vi "All GEMM.vi"() -> (3 "Benchmark":cluster{i32[], dbl[]}[](graph))   [LabVIEW 2020]
doc: "Execute GEMM Process for different size on different Toolkits (Accelerator/Culab/CUDA/LabVIEW/G2CPU) and LabVIEW(CPU)."
uses:
  <vilib>/Natan Biesmans/G2CPU GPU and CPU HPC Toolkit/ArrayFire Driver/TypeDefs/backend.ctl
  <vilib>/Natan Biesmans/G2CPU GPU and CPU HPC Toolkit/ArrayFire Driver/AF.lvlib
panel:
  out "Accelerator DirectML":bool
  out "Accelerator CUDA":bool
  out "Culab":bool
  out "Accelerator TRT":bool
  out "LabVIEW":bool
  out "G2CPU":bool
  out "Accelerator CUDA Times":dbl[](array[numeric])
  out "Accelerator CUDA Time":dbl
  out "LabVIEW Times":dbl[](array[numeric])
  out "LabVIEW Time":dbl
  out "G2CPU Times":dbl[](array[numeric])
  out "Culab Times":dbl[](array[numeric])
  out "Accelerator TRT Times":dbl[](array[numeric])
  out "G2CPU Time":dbl
  out "Culab Time":dbl
  out "Accelerator TRT Time":dbl
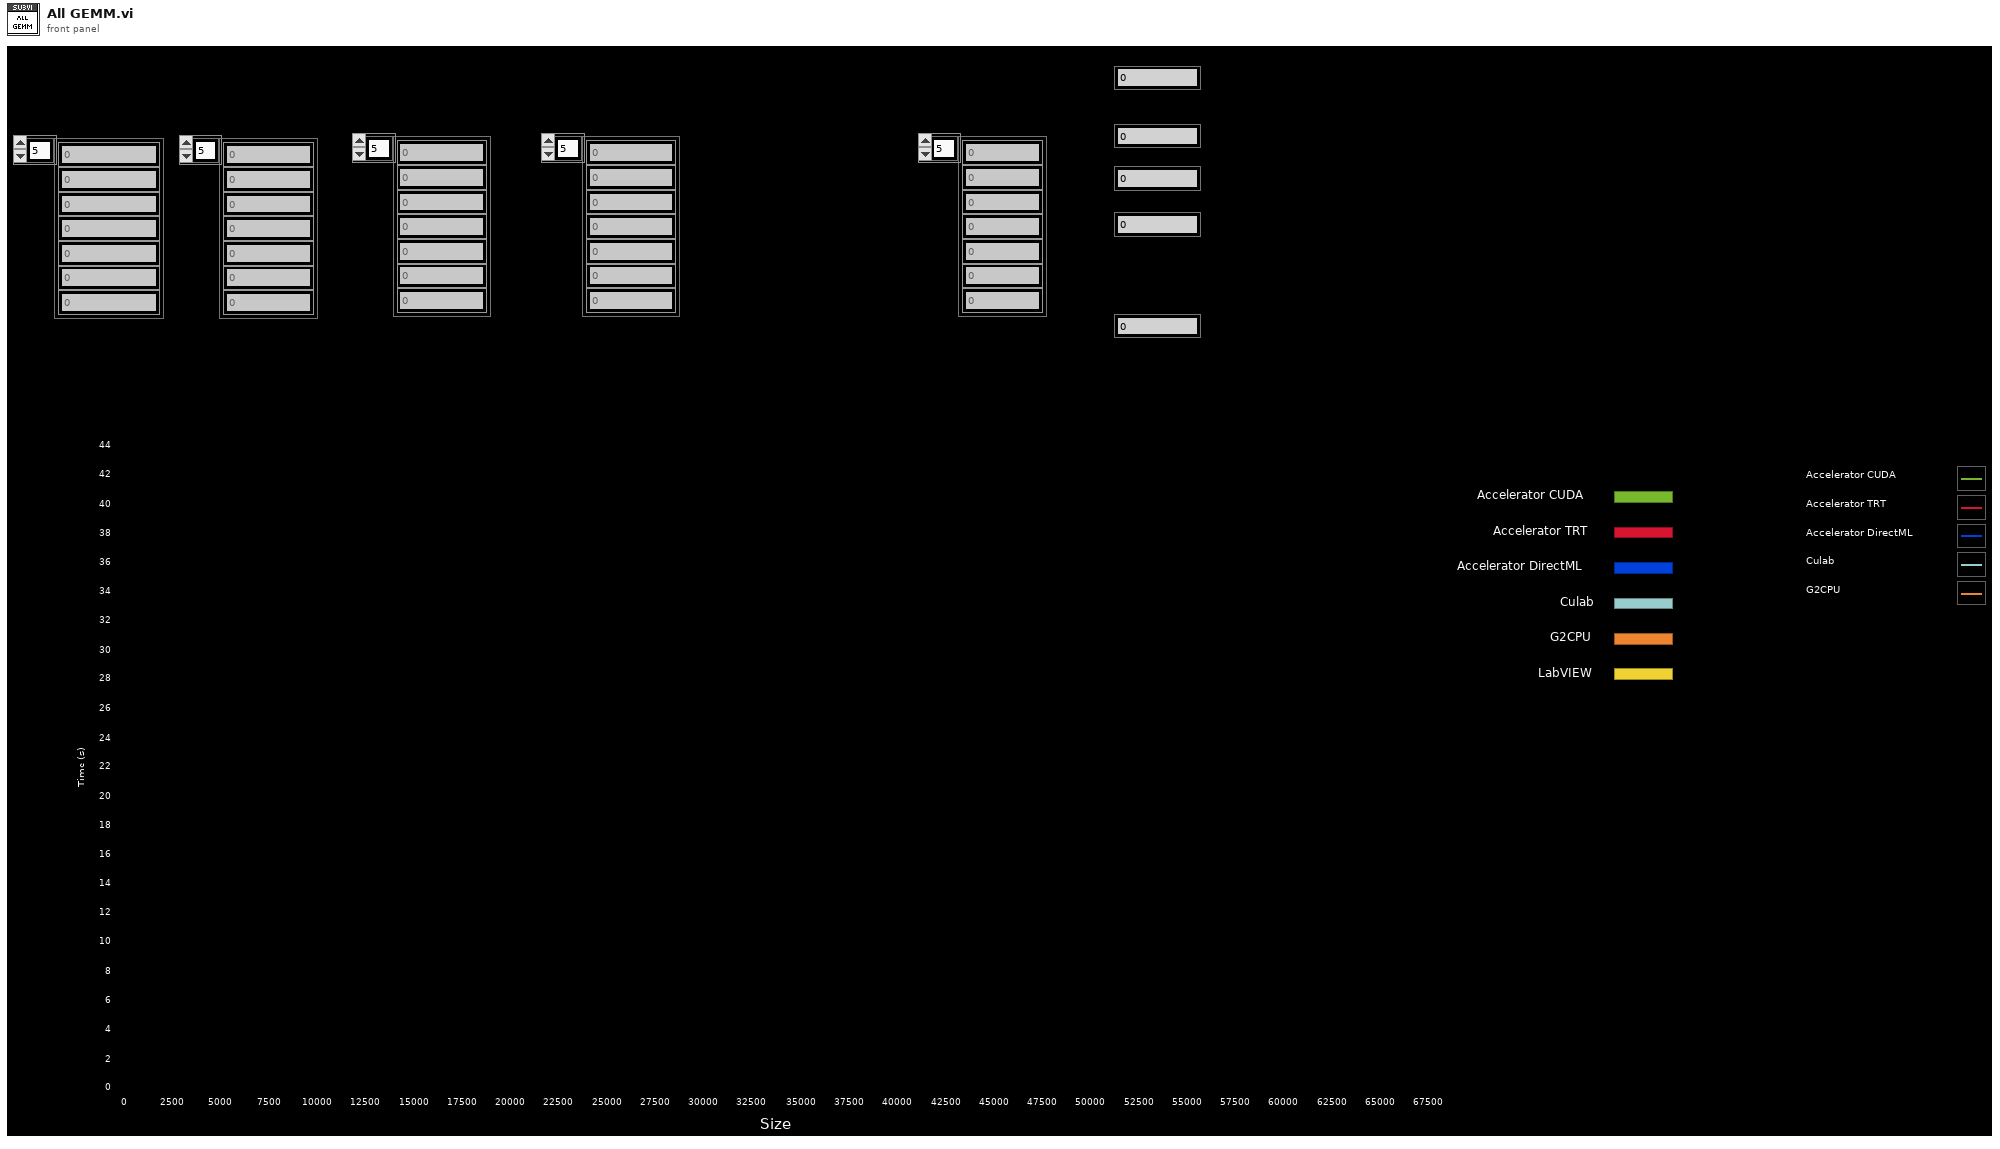
[diagram p1: front panel]
types:
  T1 = typedef "AF.lvlib/backend.ctl" = u32
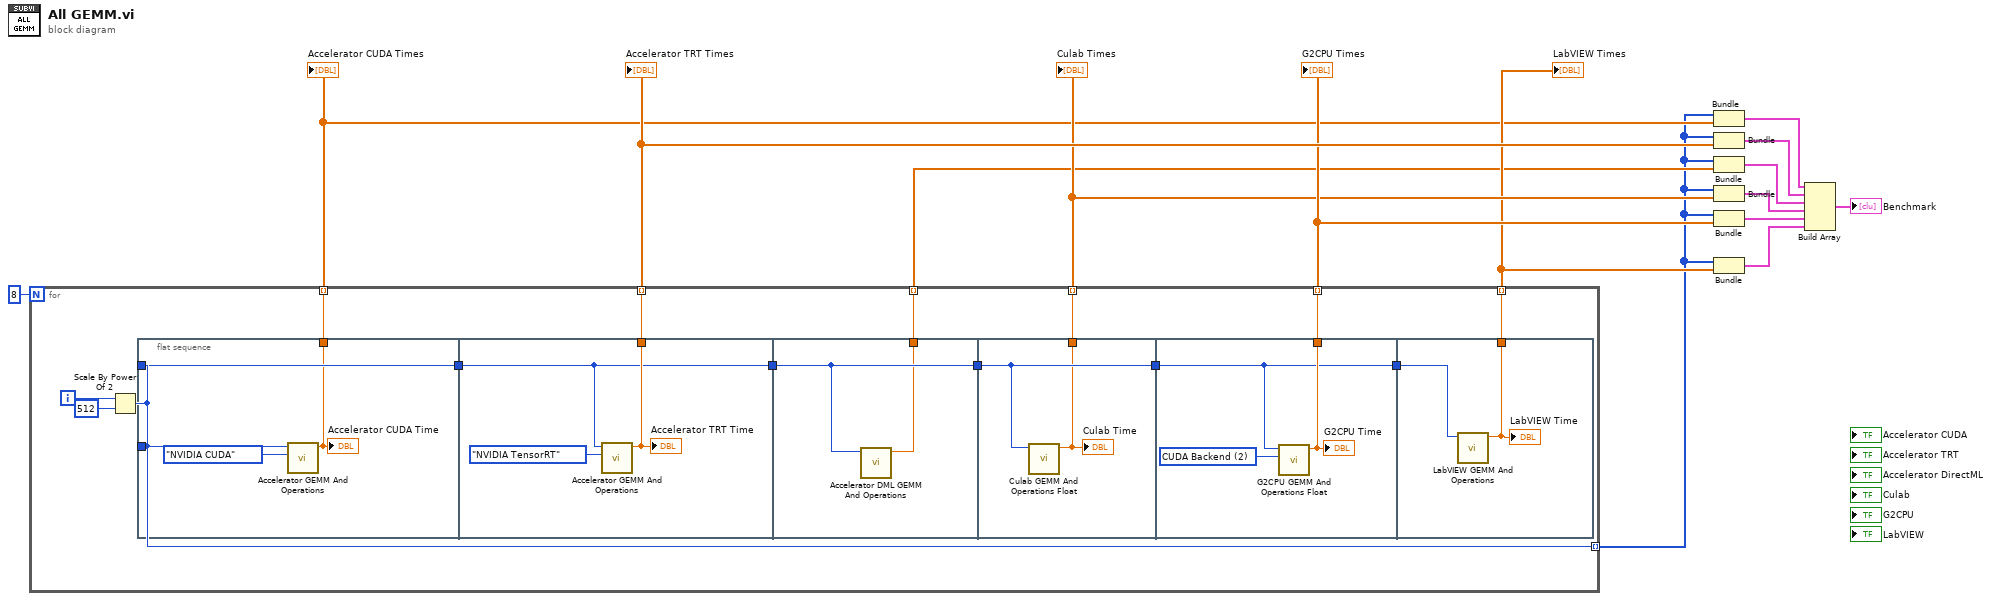
[diagram p0: block diagram]
diagram:
  n1 = for {
    N: 8 -> [_]
    tunnel: [w28] -> w14 mode=indexing
    tunnel: [w27] -> w12 mode=indexing
    tunnel: [w26] -> w13 mode=indexing
    tunnel: [w22] -> w2 mode=indexing
    tunnel: [w21] -> w9 mode=indexing
    tunnel: [w19] -> w6 mode=indexing
    tunnel: [w16] -> w3 mode=indexing
    i -> [w24]
    n2 = Scale By Power Of 2(n=w24, x=512) -> (x*2^n=w22:i32)
    n3 = flat-sequence {
      tunnel: w22 -> [w33]
      tunnel: w22 -> [w32]
      tunnel: [w33] -> w20
      tunnel: [w31] -> w19
      tunnel: [w35] -> w18
      tunnel: [w36] -> w28
      tunnel: w20 -> [w35]
      tunnel: w18 -> [w38]
      tunnel: [w38] -> w17
      tunnel: [w37] -> w16
      tunnel: w17 -> [w40]
      tunnel: [w40] -> w29
      tunnel: [w39] -> w27
      tunnel: w29 -> [w42]
      tunnel: [w43] -> w26
      tunnel: [w42] -> w23
      tunnel: [w44] -> w21
      tunnel: w23 -> [w45]
      frame #0 {
        n4 = call "Accelerator GEMM And Operations.vi"("Execution Device"=enum16{"CPU", "NVIDIA CUDA", "NVIDIA TensorRT"}."NVIDIA CUDA", "dimension size"=w32) -> ("Accelerator Time"=w31:dbl)  [unwired: 9 in]
        "Accelerator CUDA Time" <- w31
      }
      frame #1 {
        n5 = call "Accelerator GEMM And Operations.vi"("Execution Device"=enum16{"CPU", "NVIDIA CUDA", "NVIDIA TensorRT"}."NVIDIA TensorRT", "dimension size"=w35) -> ("Accelerator Time"=w36:dbl)  [unwired: 9 in]
        "Accelerator TRT Time" <- w36
      }
      frame #2 {
        n6 = call "Accelerator DML GEMM And Operations.vi"("dimension size"=w38) -> ("Accelerator Time"=w37:dbl)  [unwired: 10 in]
      }
      frame #3 {
        n7 = call "Culab GEMM And Operations Float.vi"("dimension size"=w40) -> ("Culab Time"=w39:dbl)  [unwired: 10 in]
        "Culab Time" <- w39
      }
      frame #4 {
        w41 = T1 2 items=["Default Backend"=0, "CPU Backend"=1, "CUDA Backend"=2, "OPENCL Backend"=4, "Intel OneAPI Backend"=8] ("Backend")
        n8 = call "G2CPU GEMM And Operations Float.vi"("Backend"=w41, "dimension size"=w42) -> ("G2CPU Time"=w43:dbl)  [unwired: 9 in]
        "G2CPU Time" <- w43
      }
      frame #5 {
        n9 = call "LabVIEW GEMM And Operations.vi"("dimension size"=w45) -> ("LabVIEW Time"=w44:dbl)  [unwired: 10 in]
        "LabVIEW Time" <- w44
      }
    }
  }
  "Accelerator TRT Times" <- w14
  "Culab Times" <- w12
  "G2CPU Times" <- w13
  "LabVIEW Times" <- w9
  "Accelerator CUDA Times" <- w6
  n10 = Bundle(w2, w6) -> (w7:cluster{i32[], dbl[]})  [unwired: 1 in]
  n11 = Bundle(w2, w14) -> (w8:cluster{i32[], dbl[]})  [unwired: 1 in]
  n12 = Bundle(w2, w3) -> (w1:cluster{i32[], dbl[]})  [unwired: 1 in]
  n13 = Bundle(w2, w12) -> (w11:cluster{i32[], dbl[]})  [unwired: 1 in]
  n14 = Bundle(w2, w13) -> (w10:cluster{i32[], dbl[]})  [unwired: 1 in]
  n15 = Bundle(w2, w9) -> (w5:cluster{i32[], dbl[]})  [unwired: 1 in]
  n16 = Build Array(w7, w8, w1, w11, w10, w5) -> (→"Benchmark":cluster{i32[], dbl[]}[])
